vi "Report - Excel Metadata.vi"(5 "title (\"\")":string, 6 "keywords (\"\")":string, 7 "subject (\"\")":string, 8 "error in (no error)":errorcluster, 9 "comments (\"\")":string, 10 "author (\"\")":string, 11 "NI_report in":refnum<class "NI_report.lvclass">) -> (0 "error out":errorcluster, 1 "worksheets count":i32, 2 "current worksheet name":string, 3 "NI_report out":refnum<class "NI_report.lvclass">)   [LabVIEW 2013]
uses:
  <vilib>/Utility/NIReport.llb/NI_report.lvclass
  <vilib>/Utility/NIReport.llb/Excel/NI_Excel.lvclass
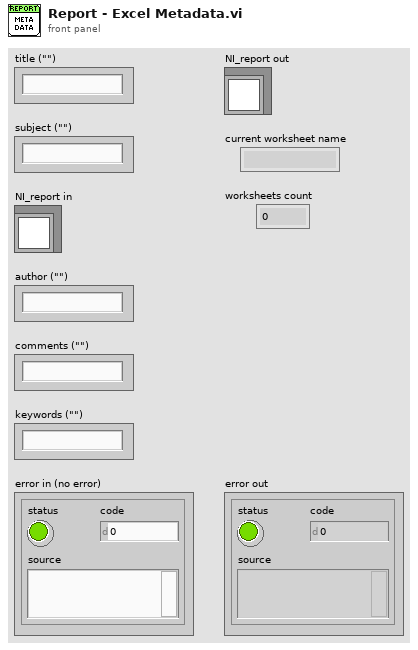
[diagram p1: front panel]
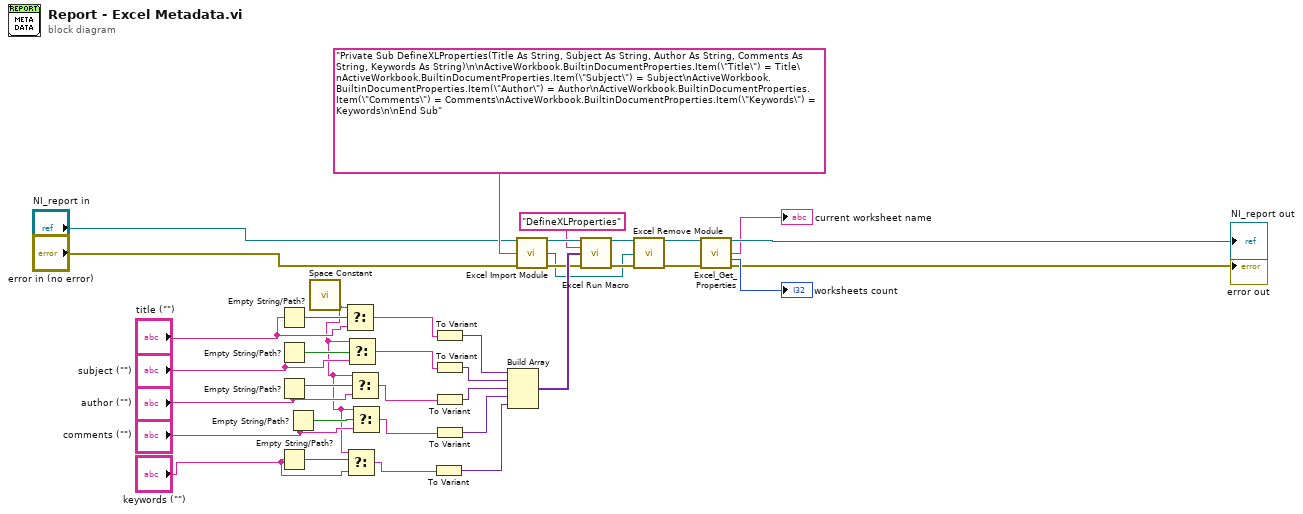
[diagram p0: block diagram]
diagram:
  n1 = Empty String/Path?(string/path="title (\"\")") -> (empty?=w16:bool)
  n2 = Empty String/Path?(string/path="subject (\"\")") -> (empty?=w12:bool)
  n3 = Empty String/Path?(string/path="author (\"\")") -> (empty?=w10:bool)
  n4 = Empty String/Path?(string/path="keywords (\"\")") -> (empty?=w4:bool)
  n5 = Empty String/Path?(string/path="comments (\"\")") -> (empty?=w7:bool)
  n6 = call <vilib>:"Space Constant.vi"() -> ("String"=w2:string)
  n7 = Select(t=w2, s=w16, f="title (\"\")") -> (s? t:f=w14:string)
  n8 = Select(t=w2, s=w4, f="keywords (\"\")") -> (s? t:f=w1:string)
  n9 = Select(t=w2, s=w12, f="subject (\"\")") -> (s? t:f=w11:string)
  n10 = Select(t=w2, s=w10, f="author (\"\")") -> (s? t:f=w8:string)
  n11 = Select(t=w2, s=w7, f="comments (\"\")") -> (s? t:f=w5:string)
  n12 = To Variant(anything=w1) -> (Variant=w37:variant)
  n13 = To Variant(anything=w14) -> (Variant=w29:variant)
  n14 = To Variant(anything=w11) -> (Variant=w31:variant)
  n15 = To Variant(anything=w8) -> (Variant=w32:variant)
  n16 = To Variant(anything=w5) -> (Variant=w30:variant)
  n17 = Build Array(w29, w31, w32, w30, w37) -> (w28:variant[])
  n18 = call <vilib>:"Excel Import Module.vi"("report in"="NI_report in", "module code (\"\")"="Private Sub DefineXLProperties(Title As String, Subject As String, Author As String, Comments As String, Keywords As String)\n\nActiveWorkbook.BuiltinDocumentProperties.Item(\"Title\") = Title\nActiveWorkbook.BuiltinDocumentProperties.Item(\"Subject\") = Subject\nActiveWorkbook.BuiltinDocumentProperties.Item(\"Author\") = Author\nActiveWorkbook.BuiltinDocumentProperties.Item(\"Comments\") = Comments\nActiveWorkbook.BuiltinDocumentProperties.Item(\"Keywords\") = Keywords\n\nEnd Sub", "error in (no error)"="error in (no error)") -> ("report out"=w20:refnum<class "NI_report.lvclass">, "module reference"=w18:refnum<k7>, "error out"=w22:errorcluster)  [unwired: 1 in, 9 out]
  n19 = call <vilib>:"Excel Run Macro.vi"("report in"=w20, "macro name"="DefineXLProperties", "parameters"=w28, "error in (no error)"=w22) -> ("report out"=w19:refnum<class "NI_report.lvclass">, "error out"=w21:errorcluster)  [unwired: 10 out]
  n20 = call <vilib>:"Excel Remove Module.vi"("report in"=w19, "module reference"=w18, "error in (no error)"=w21) -> ("report out"=w34:refnum<class "NI_report.lvclass">, "error out"=w33:errorcluster)  [unwired: 11 out]
  n21 = call <vilib>:"Excel_Get_Properties.vi"("report in"=w34, "error in (no error)"=w33) -> ("report out"=→"NI_report out":refnum<class "NI_report.lvclass">, "current worksheet name"=→"current worksheet name":string, "worksheets count"=→"worksheets count":i32, "error out"=→"error out":errorcluster)  [unwired: 10 out]
